vi "FPGAController_v6.vi"() -> ()   [LabVIEW 2015]
uses:
  Detector_Cluster.ctl
  <vilib>/Utility/miscctls.llb/LVPointTypeDef.ctl
  <vilib>/FPGAPlugInAG/PXIe-7971R/niLvFpga_Open_PXIe-7971R.vi
  <userlib>/_OpenG.lib/comparison/comparison.llb/Variant Changed__ogtk.vi
  <vilib>/Utility/error.llb/Error Cluster From Error Code.vi
  <vilib>/rvi/errors/niLvFpgaAdjustHostInterfaceError.vi
  <vilib>/FPGAPlugInAG/PXIe-7971R/niLvFpga_Close_PXIe-7971R.vi
  <vilib>/rvi/interface/nirviOpenFPGA/nirviOpenFPGA.xnode
  FPGA Bitfiles/FPGA2_FPGATarget_FPGAcode2_Gw4Ab0yitnw.lvbitx
  <vilib>/rvi/interface/nirviReadWriteControl/nirviReadWriteControl.xnode
  Limits_In.ctl
  <vilib>/rvi/interface/nirviCloseFPGA/nirviCloseFPGA.xnode
  NiFpgaLv.dll
panel:
  in  "Trigger String 2":string="Disarm FPGA"
  in  "Trigger String 1":string="Rearm FPGA"
  in  "Tab Control":enum32{"IO/Control", "Error Management"}(tab)
  out "FPGA Armed":bool=TRUE
  in  "Arm FPGA":bool
  in  "One Shot Mode":bool
  in  "Auto Threshold":bool
  in  "Sensitivity":dbl=1.2 step=0.2 format="%_3g"
  in  "Filter Thresholds":T1={"1"=887988, "2"=361992, "3"=138762, "4"=54306, "5"=41730, "6"=29358, "7"=21165}
  in  "error in (no error)":errorcluster
  out "error out":errorcluster
  out "Runtime Error":errorcluster
  out "Updating PSU":bool
  in  "stop":bool
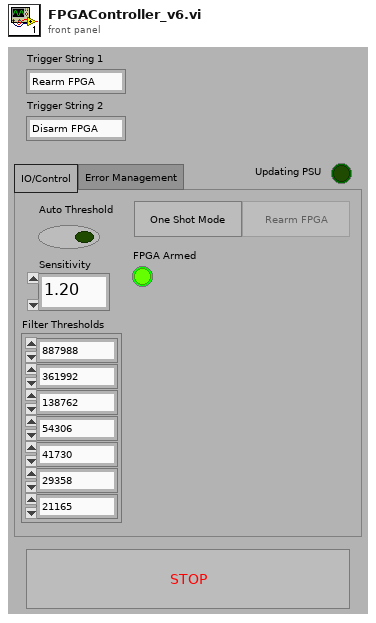
[diagram p1: front panel]
types:
  T1 = typedef "Detector_Cluster.ctl" = cluster{"1":i32, "2":i32, "3":i32, "4":i32, "5":i32, "6":i32, "7":i32}
  T2 = enum8{"Enabled", "Disabled", "Disabled and Grayed Out"}
  T3 = typedef "LVPointTypeDef.ctl" = cluster{"Horizontal":i16, "Vertical":i16}
  T4 = typedef "Limits_In.ctl" = cluster{"High Charge Limit":i16, "Low Charge Limit":i16, "High Velocity Count":i32, "Low Velocity Count":i32, "High Mass Limit":i64, "Low Mass Limit":i64}
  T5 = cluster{"1":dbl, "2":dbl, "3":dbl, "4":dbl, "5":dbl, "6":dbl, "7":dbl}
  T6 = cluster{"1":i16, "2":i16, "3":i16, "4":i16, "5":i16, "6":i16, "7":i16}
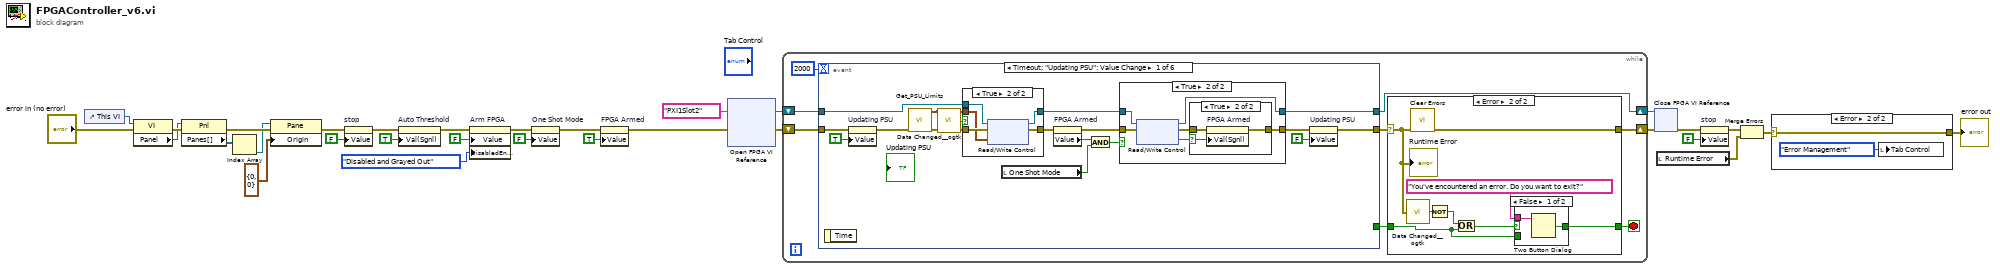
[diagram p0: block diagram]
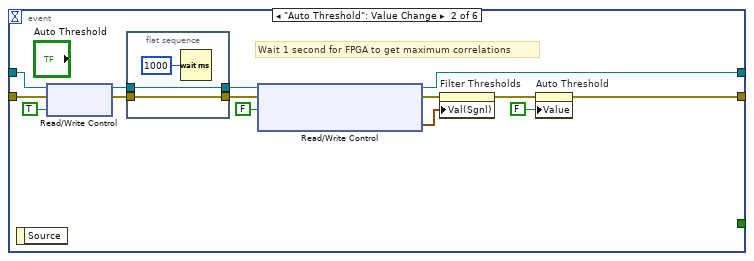
[diagram p8: hidden frame]
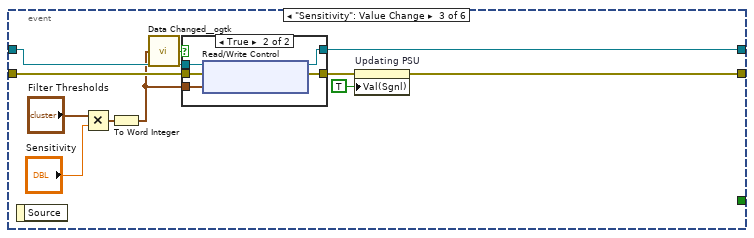
[diagram p9: hidden frame]
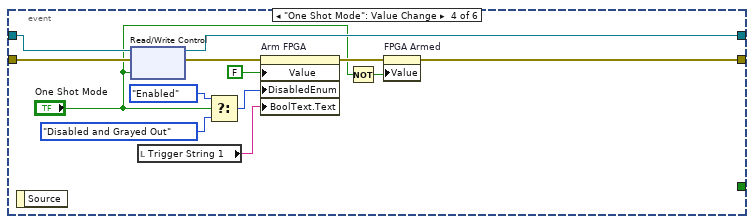
[diagram p11: hidden frame]
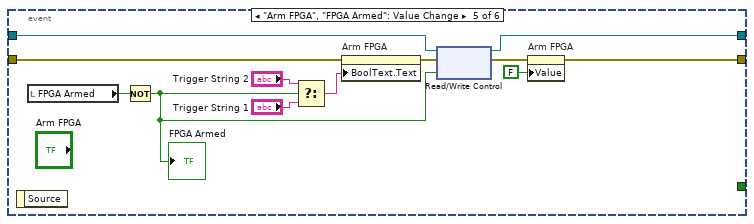
[diagram p12: hidden frame]
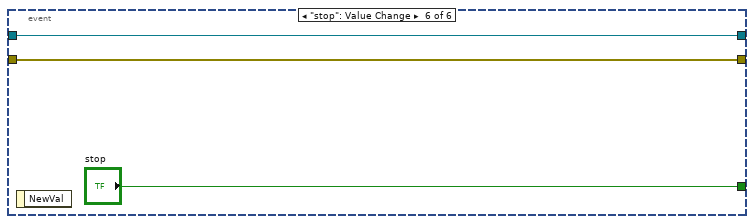
[diagram p13: hidden frame]
diagram:
  n1 = control-ref of="This VI"() -> (w31:refnum<vi>)
  n2 = property class="VI"(reference=w31, error in="error in (no error)") -> (error out=w30:errorcluster, "Panel"=w29:refnum<vi>)  [unwired: 1 out]
  n3 = property class="Pnl"(reference=w29, error in=w30) -> (error out=w28:errorcluster, "Panes[]"=w27:refnum<vi>[])  [unwired: 1 out]
  n4 = Index Array(array=w27) -> (element=w26:refnum<vi>)  [unwired: 1 in]
  n5 = property class="Pane"(reference=w26, error in=w28, "Origin"=T3 {"Horizontal"=0, "Vertical"=0}) -> (error out=w19:errorcluster)  [unwired: 1 out]
  n6 = property on="stop" class="Bool (strict)"(error in=w19, "Value"=FALSE ("stop")) -> (error out=w15:errorcluster)  [unwired: 1 in, 1 out]
  n7 = property on="Auto Threshold" class="Bool (strict)"(error in=w15, "Val(Sgnl)"=TRUE ("Value (Signaling)")) -> (error out=w7:errorcluster)  [unwired: 1 in, 1 out]
  n8 = property on="Arm FPGA" class="Bool (strict)"(error in=w7, "Value"=FALSE ("Arm Trigger"), "DisabledEnum"=T2."Disabled and Grayed Out" ("Disabled")) -> (error out=w5:errorcluster)  [unwired: 1 in, 1 out]
  n9 = property on="One Shot Mode" class="Bool (strict)"(error in=w5, "Value"=FALSE ("One Shot Mode")) -> (error out=w3:errorcluster)  [unwired: 1 in, 1 out]
  n10 = property on="FPGA Armed" class="Bool (strict)"(error in=w3, "Value"=TRUE ("Armed")) -> (error out=w1:errorcluster)  [unwired: 1 in, 1 out]
  n11 = xnode "Open FPGA VI Reference"("error in"=w1, "resource name"=tag "PXI1Slot2") -> ("FPGA VI Reference Out"=w23:refnum<k20>, "error out"=w21:errorcluster)
  n12 = while {
    shift-right: [w32] -> w20
    shift-left: w21 -> [w38]
    shift-right: [w36] -> w22
    shift-left: w23 -> [w37]
    stop <- w34 stop-if-true
    n13 = event shown="[0] Timeout;  \"Updating PSU\": Value Change" {
      selector: _ -> [_ _ _ _ _ _]
      dyn-events: _ -> [_ _ _ _ _ _]
      timeout: 2000 -> [_ _ _ _ _ _]
      tunnel: [_ _ _ _ _ "stop"] -> w33
      tunnel: w38 -> [w67 w100 w115 w136 w148 w150]
      tunnel: [w61 w102 w109 w126 w138 w150] -> w35
      tunnel: w37 -> [w69 w99 w116 w135 w143 w149]
      tunnel: [w56 w94 w112 w129 w142 w149] -> w36
      event Timeout; "Updating PSU": Value Change {
        n14 = event-data() -> ()  [unwired: 1 in, 1 out]
        n15 = property on="Updating PSU" class="Bool (strict)"(error in=w67, "Value"=TRUE ("Updating PSU")) -> (error out=w64:errorcluster)  [unwired: 1 in, 1 out]
        n16 = call "Get_PSU_Limits.vi"("error in (no error)"=w64) -> ("error out"=w68:errorcluster, "Limits"=w63:T4)  [unwired: 9 in]
        n17 = call-poly <userlib>:"Data Changed__ogtk.vi"("Variant"=w63) -> ("Changed"=w62:bool)
        n18 = case shown="True" w62 {
          tunnel: w69 -> [w83 w88]
          tunnel: w68 -> [w82 w87]
          tunnel: [w83 w86] -> w57
          tunnel: [w82 w85] -> w60
          tunnel: w63 -> [_ w84]
          frame False {
          }
          frame True {
            n19 = xnode "Read/Write Control"("FPGA VI Reference In"=w88, "error in"=w87, "Limits"=w84) -> ("FPGA VI Reference Out"=w86:refnum<k20>, "error out"=w85:errorcluster)
          }
        }
        n20 = local read "One Shot Mode"() -> (w53:bool)
        n21 = property on="FPGA Armed" class="Bool (strict)"(error in=w60) -> (error out=w58:errorcluster, "Value"=w59:bool)  [unwired: 1 in, 1 out]
        n22 = And(x=w59, y=w53) -> (x .and. y?=w54:bool)
        n23 = case shown="True" w54 {
          tunnel: w58 -> [w70 w77]
          tunnel: w57 -> [w71 w76]
          tunnel: [w71 w75] -> w56
          tunnel: [w70 w73] -> w55
          frame False {
          }
          frame True {
            n24 = xnode "Read/Write Control"("FPGA VI Reference In"=w76, "error in"=w77) -> ("FPGA VI Reference Out"=w75:refnum<k20>, "error out"=w74:errorcluster, "Armed"=w72:bool)
            n25 = case shown="True" w72 {
              selector: w72 -> [_ w79]
              tunnel: w74 -> [w78 w81]
              tunnel: [w78 w80] -> w73
              frame False {
              }
              frame True {
                n26 = property on="FPGA Armed" class="Bool (strict)"(error in=w81, "Val(Sgnl)"=w79) -> (error out=w80:errorcluster)  [unwired: 1 in, 1 out]
              }
            }
          }
        }
        n27 = property on="Updating PSU" class="Bool (strict)"(error in=w55, "Value"=FALSE ("Updating PSU")) -> (error out=w61:errorcluster)  [unwired: 1 in, 1 out]
      }
      event "Auto Threshold": Value Change {
        # "Wait 1 second for FPGA to get maximum correlations"
        n28 = event-data() -> ()  [unwired: 1 in, 1 out]
        n29 = xnode "Read/Write Control"("FPGA VI Reference In"=w99, "error in"=w100, "Calibrate"=TRUE) -> ("FPGA VI Reference Out"=w97:refnum<k20>, "error out"=w98:errorcluster)
        n30 = flat-sequence {
          tunnel: w98 -> [w103]
          tunnel: w97 -> [w104]
          tunnel: [w104] -> w96
          tunnel: [w103] -> w95
          frame #0 {
            n31 = Wait (ms)(milliseconds to wait=u32 1000) -> ()  [unwired: 1 out]
          }
        }
        n32 = xnode "Read/Write Control"("FPGA VI Reference In"=w96, "error in"=w95, "Calibrate"=FALSE) -> ("FPGA VI Reference Out"=w94:refnum<k20>, "error out"=w90:errorcluster, "Detector 3 Max Correlations"=w91:T1)
        n33 = property on="Filter Thresholds" class="Clust (strict)"(error in=w90, "Val(Sgnl)"=w91) -> (error out=w89:errorcluster)  [unwired: 1 in, 1 out]
        n34 = property on="Auto Threshold" class="Bool (strict)"(error in=w89, "Value"=FALSE ("Auto Threshold")) -> (error out=w102:errorcluster)  [unwired: 1 in, 1 out]
      }
      event "Sensitivity": Value Change {
        n35 = event-data() -> ()  [unwired: 1 in, 1 out]
        n36 = Multiply(x="Filter Thresholds", y="Sensitivity") -> (x*y=w114:T5)
        n37 = To Word Integer(number=w114) -> (16bit integer=w106:T6)
        n38 = call-poly <userlib>:"Data Changed__ogtk.vi"("Variant"=w106) -> ("Changed"=w107:bool)
        n39 = case shown="True" w107 {
          tunnel: w116 -> [w117 w123]
          tunnel: w115 -> [w118 w122]
          tunnel: [w117 w121] -> w112
          tunnel: [w118 w120] -> w110
          tunnel: w106 -> [_ w119]
          frame False {
          }
          frame True {
            n40 = xnode "Read/Write Control"("FPGA VI Reference In"=w123, "error in"=w122, "Filter Thresholds"=w119) -> ("FPGA VI Reference Out"=w121:refnum<k20>, "error out"=w120:errorcluster)
          }
        }
        n41 = property on="Updating PSU" class="Bool (strict)"(error in=w110, "Val(Sgnl)"=TRUE ("Updating PSU")) -> (error out=w109:errorcluster)  [unwired: 1 in, 1 out]
      }
      event "One Shot Mode": Value Change {
        n42 = event-data() -> ()  [unwired: 1 in, 1 out]
        n43 = xnode "Read/Write Control"("FPGA VI Reference In"=w135, "error in"=w136, "Armed"="One Shot Mode") -> ("FPGA VI Reference Out"=w129:refnum<k20>, "error out"=w133:errorcluster)
        n44 = local read "Trigger String 1"() -> (w128:string)
        n45 = Select(t=T2."Enabled" ("Disabled"), s="One Shot Mode", f=T2."Disabled and Grayed Out" ("Disabled")) -> (s? t:f=w132:T2)
        n46 = property on="Arm FPGA" class="Bool (strict)"(error in=w133, "Value"=FALSE ("Arm Trigger"), "DisabledEnum"=w132, "BoolText.Text"=w128) -> (error out=w127:errorcluster)  [unwired: 1 in, 1 out]
        n47 = Not(x="One Shot Mode") -> (.not. x?=w125:bool)
        n48 = property on="FPGA Armed" class="Bool (strict)"(error in=w127, "Value"=w125) -> (error out=w126:errorcluster)  [unwired: 1 in, 1 out]
      }
      event "Arm FPGA", "FPGA Armed": Value Change {
        n49 = event-data() -> ()  [unwired: 1 in, 1 out]
        n50 = local read "FPGA Armed"() -> (w141:bool)
        n51 = Not(x=w141) -> (.not. x?=w140:bool)
        "FPGA Armed" <- w140
        n52 = Select(t="Trigger String 2", s=w140, f="Trigger String 1") -> (s? t:f=w145:string)
        n53 = property on="Arm FPGA" class="Bool (strict)"(error in=w148, "BoolText.Text"=w145) -> (error out=w144:errorcluster)  [unwired: 1 in, 1 out]
        n54 = xnode "Read/Write Control"("FPGA VI Reference In"=w143, "error in"=w144, "Armed"=w140) -> ("FPGA VI Reference Out"=w142:refnum<k20>, "error out"=w139:errorcluster)
        n55 = property on="Arm FPGA" class="Bool (strict)"(error in=w139, "Value"=FALSE ("Arm Trigger")) -> (error out=w138:errorcluster)  [unwired: 1 in, 1 out]
      }
      event "stop": Value Change {
        n56 = event-data() -> ()  [unwired: 1 in, 1 out]
      }
    }
    n57 = case shown="Error" w35 {
      selector: w35 -> [w41 w46]
      tunnel: [w41 w49] -> w32
      tunnel: [w40 w47] -> w34
      tunnel: w33 -> [w40 w42]
      frame No Error {
      }
      frame Error {
        n58 = call-poly <userlib>:"Data Changed__ogtk.vi"("Variant"=w46) -> ("Changed"=w44:bool)
        n59 = call <vilib>:"Clear Errors.vi"("error in (no error)"=w46) -> ("error out"=w49:errorcluster)  [unwired: 5 in, 1 out]
        n60 = Not(x=w44) -> (.not. x?=w43:bool)
        n61 = Or(x=w43, y=w42) -> (x .or. y?=w45:bool)
        n62 = case shown="False" w45 {
          tunnel: "You've encountered an error. Do you want to exit?" ("message") -> [w51 _]
          tunnel: [w50 w52] -> w47
          tunnel: w42 -> [_ w52]
          frame False {
            n63 = Two Button Dialog(message=w51) -> (T button?=w50:bool)  [unwired: 2 in]
          }
          frame True {
          }
        }
        "Runtime Error" <- w46
      }
    }
  }
  n64 = xnode "Close FPGA VI Reference"("FPGA VI Reference In"=w22, "error in"=w20) -> ("error out"=w16:errorcluster)
  n65 = local read "Runtime Error"() -> (w11:errorcluster)
  n66 = property on="stop" class="Bool (strict)"(error in=w16, "Value"=FALSE ("stop")) -> (error out=w12:errorcluster)  [unwired: 1 in, 1 out]
  n67 = Merge Errors(w12, w11) -> (w9:errorcluster)
  n68 = case shown="Error" w9 {
    selector: w9 -> [w152 w153]
    tunnel: [w152 w153] -> w10
    frame No Error {
    }
    frame Error {
      n69 = local write "Tab Control"(enum32{"IO/Control", "Error Management"}."Error Management" ("Tab Control")) -> ()
    }
  }
  "error out" <- w10
